vi "Configure Multiple Baseband Generator Synchronization.vi"(6 "Slave Position (1)":i32=1, 8 "error in (no error)":errorcluster, 9 "Number Of Slaves (1)":i32=1, 10 "Multiple BBG Synchronization Setup (0: Off)":u16(ring) items=["Off", "Master", "Slave"], 11 "VISA resource name":refnum<visa-resource-name>) -> (0 "error out":errorcluster, 3 "VISA resource name out":refnum<visa-resource-name>)   [LabVIEW 2011, in "Agilent PSG MXG Series.lvlib"]
doc: "Configures the multiple BBG synchronization setup.\n\n<B>Notes:</B>\n(1) This VI is valid only in N5182A that installs <B>Option 651</B> or <B>Option 652</B> or <B>Option 654</B> (Internal baseband generator)."
uses:
  Agilent PSG MXG Series.lvlib
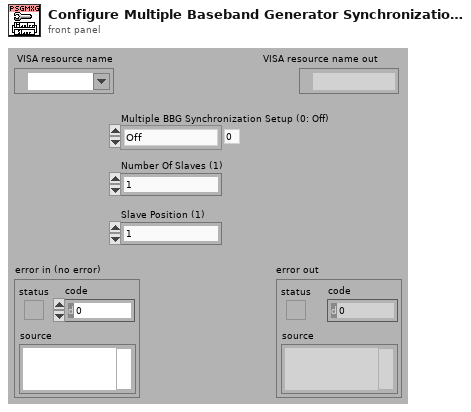
[diagram p1: front panel]
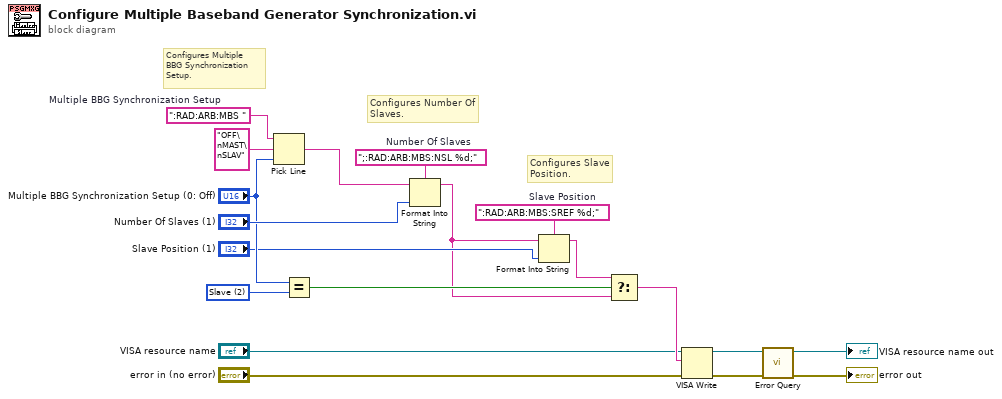
[diagram p0: block diagram]
diagram:
  w12 = ":RAD:ARB:MBS:SREF %d;"  # Slave Position
  w13 = u16 2 items=["Off", "Master", "Slave"] ("Multiple BBG Synchronization Setup (0: Off)")
  w16 = ";:RAD:ARB:MBS:NSL %d;"  # Number Of Slaves
  w18 = ":RAD:ARB:MBS "  # Multiple BBG Synchronization Setup
  # "Configures Slave\nPosition."
  # "Configures Number Of\nSlaves."
  # "Configures Multiple\nBBG Synchronization\nSetup."
  n1 = Pick Line(string ("")=w18, multi-line string="OFF\nMAST\nSLAV", line index="Multiple BBG Synchronization Setup (0: Off)") -> (output string=w17:string)
  n2 = Equal?(x="Multiple BBG Synchronization Setup (0: Off)", y=w13) -> (x = y?=w10:bool)
  n3 = Format Into String(format string=w16, initial string=w17, "Number Of Slaves (1)") -> (resulting string=w8:string)  [unwired: 1 in, 1 out]
  n4 = Format Into String(format string=w12, initial string=w8, "Slave Position (1)") -> (resulting string=w9:string)  [unwired: 1 in, 1 out]
  n5 = Select(t=w9, s=w10, f=w8) -> (s? t:f=w7:string)
  n6 = VISA Write(VISA resource name="VISA resource name", write buffer=w7, error in (no error)="error in (no error)") -> (VISA resource name out=w6:refnum<visa-resource-name>, error out=w5:errorcluster)  [unwired: 1 out]
  n7 = call "Error Query.vi"("error in (no error)"=w5, "VISA resource name"=w6) -> ("error out"=→"error out":errorcluster, "VISA resource name out"=→"VISA resource name out":refnum<visa-resource-name>)  [unwired: 6 in, 2 out]
